vi "Map reset.vi"(2 "i":i64) -> (6 "MAP":T1)   [LabVIEW 2010]
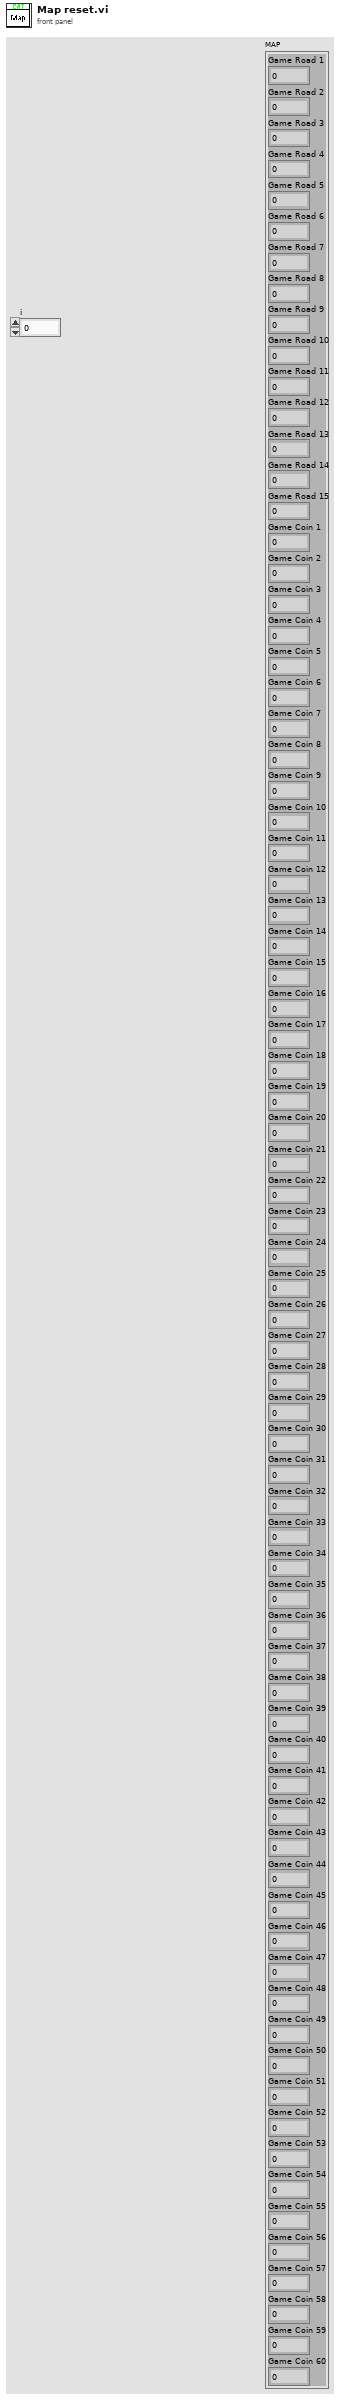
[diagram p1: front panel]
types:
  T1 = cluster{"Game Road 1":u16, "Game Road 2":u16, "Game Road 3":u16, "Game Road 4":u16, "Game Road 5":u16, "Game Road 6":u16, "Game Road 7":u16, "Game Road 8":u16, "Game Road 9":u16, "Game Road 10":u16, "Game Road 11":u16, "Game Road 12":u16, "Game Road 13":u16, "Game Road 14":u16, "Game Road 15":u16, "Game Coin 1":u16, "Game Coin 2":u16, "Game Coin 3":u16, "Game Coin 4":u16, "Game Coin 5":u16, "Game Coin 6":u16, "Game Coin 7":u16, "Game Coin 8":u16, "Game Coin 9":u16, "Game Coin 10":u16, "Game Coin 11":u16, "Game Coin 12":u16, "Game Coin 13":u16, "Game Coin 14":u16, "Game Coin 15":u16, "Game Coin 16":u16, "Game Coin 17":u16, "Game Coin 18":u16, "Game Coin 19":u16, "Game Coin 20":u16, "Game Coin 21":u16, "Game Coin 22":u16, "Game Coin 23":u16, "Game Coin 24":u16, "Game Coin 25":u16, "Game Coin 26":u16, "Game Coin 27":u16, "Game Coin 28":u16, "Game Coin 29":u16, "Game Coin 30":u16, "Game Coin 31":u16, "Game Coin 32":u16, "Game Coin 33":u16, "Game Coin 34":u16, "Game Coin 35":u16, "Game Coin 36":u16, "Game Coin 37":u16, "Game Coin 38":u16, "Game Coin 39":u16, "Game Coin 40":u16, "Game Coin 41":u16, "Game Coin 42":u16, "Game Coin 43":u16, "Game Coin 44":u16, "Game Coin 45":u16, "Game Coin 46":u16, "Game Coin 47":u16, "Game Coin 48":u16, "Game Coin 49":u16, "Game Coin 50":u16, "Game Coin 51":u16, "Game Coin 52":u16, "Game Coin 53":u16, "Game Coin 54":u16, "Game Coin 55":u16, "Game Coin 56":u16, "Game Coin 57":u16, "Game Coin 58":u16, "Game Coin 59":u16, "Game Coin 60":u16}
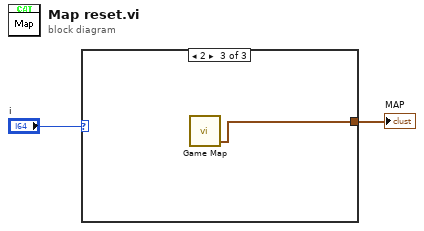
[diagram p0: block diagram]
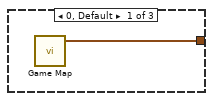
[diagram p2: hidden frame]
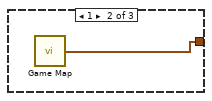
[diagram p3: hidden frame]
diagram:
  n1 = case shown="2" "i" {
    tunnel: [w3 w4 w5] -> w1
    frame 0, Default {
      n2 = call "Game Map.vi"() -> ("MAP1"=w3:T1)  [unwired: 5 in, 2 out]
    }
    frame 1 {
      n3 = call "Game Map.vi"() -> ("MAP2"=w4:T1)  [unwired: 5 in, 2 out]
    }
    frame 2 {
      n4 = call "Game Map.vi"() -> ("MAP3"=w5:T1)  [unwired: 5 in, 2 out]
    }
  }
  "MAP" <- w1
